vi "LPS Example.vi"() -> ()   [LabVIEW 2020]
doc: "Example for reading from the LPS pressure/temperature/altitude (barometer) sensor using the LINX toolkit."
uses:
  <vilib>/MakerHub/LINX/Public/Utilities/Open Local.vi
  LINX I2C/LINX I2C.lvclass
  LPS Barometric Pressure/LPS Barometric Pressure Sensor.lvclass
  <vilib>/MakerHub/LINX/LMH-LINX.lvlib
panel:
  in  "stop":bool
  out "Waveform Chart":dbl[][](graph)
  out "Error Out":errorcluster
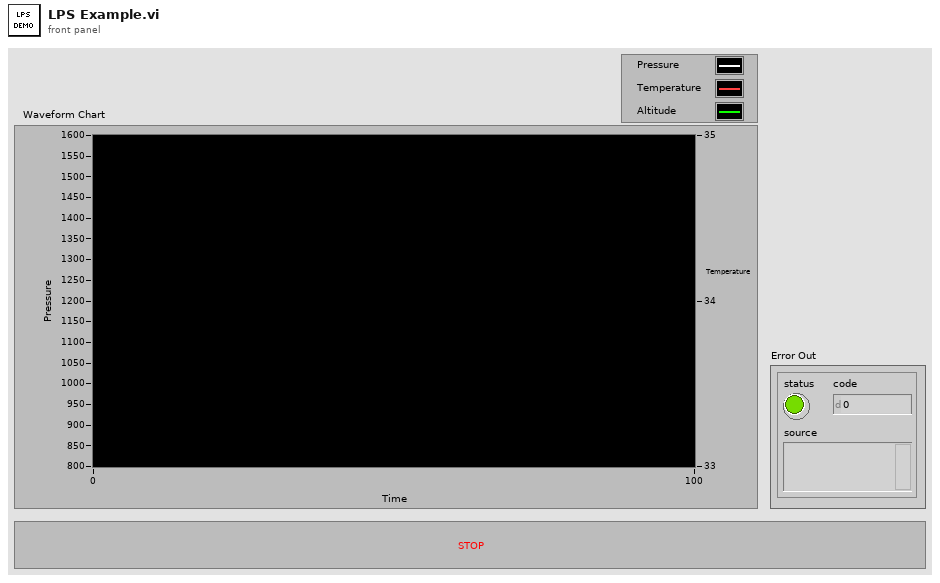
[diagram p1: front panel]
types:
  T1 = typedef "LMH-LINX.lvlib/LINX Ref.ctl" = cluster{"IO":T2, "Interface":T3, "LINX Device Config":T4}
  T2 = typedef "LMH-LINX.lvlib/Platform.ctl" = enum16{"Remote", "Local"}
  T3 = typedef "LMH-LINX.lvlib/Interface.ctl" = enum16{"Serial", "TCP"}
  T4 = typedef "LMH-LINX.lvlib/Device.lvlib/LINX Device Config.ctl" = cluster{"Interface":T3, "COM Port":refnum<visa-resource-name>, "TCP Configuration":T5, "Device Family":u8, "Device ID":u8, "Device Name":string, "TCP Ref":refnum<k5>, "Channels":T6}
  T5 = typedef "LMH-LINX.lvlib/Device.lvlib/TCP Config.ctl" = cluster{"IP Address":string, "Port":u16}
  T6 = typedef "LMH-LINX.lvlib/Channels.ctl" = cluster{"DI":u8[], "DO":u8[], "AI":u8[], "AO":u8[], "PWM":u8[], "QE":u8[], "UART":u8[], "I2C 2":u8[], "SPI":u8[], "CAN":u8[], "Servo":u8[], "AI Ref (V)":dbl, "AI Resolution (Bits)":u8, "AO Ref (V)":dbl, "AO Resolution (Bits)":u8}
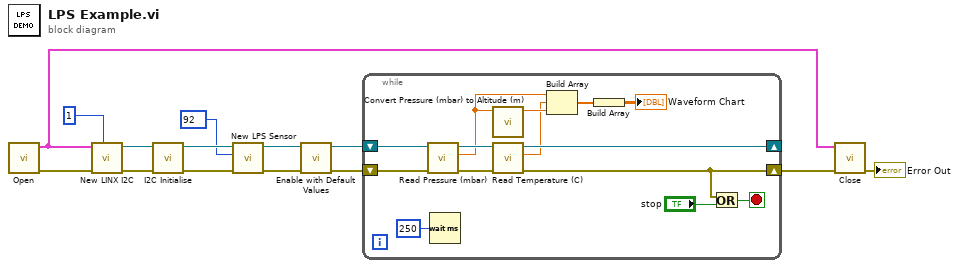
[diagram p0: block diagram]
diagram:
  n1 = call-poly <vilib>:"Open.vi"() -> ("Error Out"=w13:errorcluster, "LINX Resource"=w9:T1)  [unwired: 9 in, 1 out]
  n2 = call "New LINX I2C.vi"("LINX I2C Channel"=u8 1 ("I2C Channel"), "error in (no error)"=w13, "LINX Resource"=w9) -> ("error out"=w11:errorcluster, "LINX I2C out"=w10:refnum<class "LINX I2C.lvclass">)  [unwired: 7 in]
  n3 = call-dynamic "I2C Initialise.vi"("error in (no error)"=w11, "LINX I2C in"=w10) -> ("error out"=w8:errorcluster, "LINX I2C out"=w7:refnum<class "LINX I2C.lvclass">)  [unwired: 8 in]
  n4 = call "New LPS Sensor.vi"("error in (no error)"=w8, "I2C Slave Address (0x5D)"=u8 92, "I2C"=w7) -> ("error out"=w5:errorcluster, "LPS Barometer out"=w4:refnum<class "LPS Barometric Pressure Sensor.lvclass">)  [unwired: 7 in]
  n5 = call-dynamic "Enable with Default Values.vi"("error in (no error)"=w5, "LPS Barometer in"=w4) -> ("error out"=w3:errorcluster, "LPS Barometer out"=w2:refnum<class "LPS Barometric Pressure Sensor.lvclass">)  [unwired: 8 in]
  n6 = while {
    shift-right: [w20] -> w1
    shift-left: w3 -> [w28]
    shift-right: [w22] -> _
    shift-left: w2 -> [w27]
    stop <- w24 stop-if-true
    n7 = call "Read Pressure (mbar).vi"("error in (no error)"=w28, "LPS Barometric Pressure Sensor in"=w27) -> ("error out"=w21:errorcluster, "Pressure (mbar/hPa)"=w17:dbl, "LPS Barometric Pressure Sensor out"=w26:refnum<class "LPS Barometric Pressure Sensor.lvclass">)  [unwired: 7 in]
    n8 = Wait (ms)(milliseconds to wait=u32 250) -> ()  [unwired: 1 out]
    n9 = call "Convert Pressure (mbar) to Altitude (m).vi"("Pressure (mbar)"=w17) -> ("Altitude (m)"=w16:dbl)  [unwired: 10 in]
    n10 = call "Read Temperature (C).vi"("error in (no error)"=w21, "LPS Barometric Pressure Sensor in"=w26) -> ("error out"=w20:errorcluster, "Temperature (degC)"=w15:dbl, "LPS Barometric Pressure Sensor out"=w22:refnum<class "LPS Barometric Pressure Sensor.lvclass">)  [unwired: 7 in]
    n11 = Build Array(w17, w15, w16) -> (w19:dbl[])
    n12 = Build Array(w19) -> (→"Waveform Chart":dbl[][])
    n13 = Or(x=w20, y="stop") -> (x .or. y?=w24:bool)
  }
  n14 = call <vilib>:"Close.vi"("Error In"=w1, "LINX Resource"=w9) -> ("Error Out"=→"Error Out":errorcluster)  [unwired: 9 in]
